vi "CODMn通讯.vi"() -> ()   [LabVIEW 2016, in "斯坦道CODMn.lvlib"]
uses:
  <vilib>/NI/Modbus Library/API/Wrapper/Create TCP Slave.vi
  <vilib>/NI/Modbus Library/API/slave/Modbus Slave.lvclass
  <vilib>/Plasmionique/MB Master/MB_Master/MB_Master.lvclass
  <vilib>/Plasmionique/MB Master/MB Master.lvlib
  <vilib>/NI/Modbus Library/API/Wrapper/API Main.lvlib
  <vilib>/ptbypt/NI_PtbyPt.lvlib
panel:
  out "F0-F5":u16[](array[numeric])
  out "codm程序更新":bool=TRUE
  in  "读取数据":bool
  in  "释放串口":bool
  in  "打开串口":bool
  out "队列中元素数量":i32
  out "元素":cluster{"命令":string}[](array[cluster])
  out "待处理插入数量":i32
  out "读取公式":u16[](array[numeric])
  out "读取参数":u16[](array[numeric])
  out "数据存储":u16[](array[numeric])
  out "温度":bool[](array[boolean])
  out "M输出点":bool[](array[boolean])
  out "ORP、时间":u16[](array[numeric])
  out "测量状态":u16[](array[numeric])
  out "通讯状态":bool
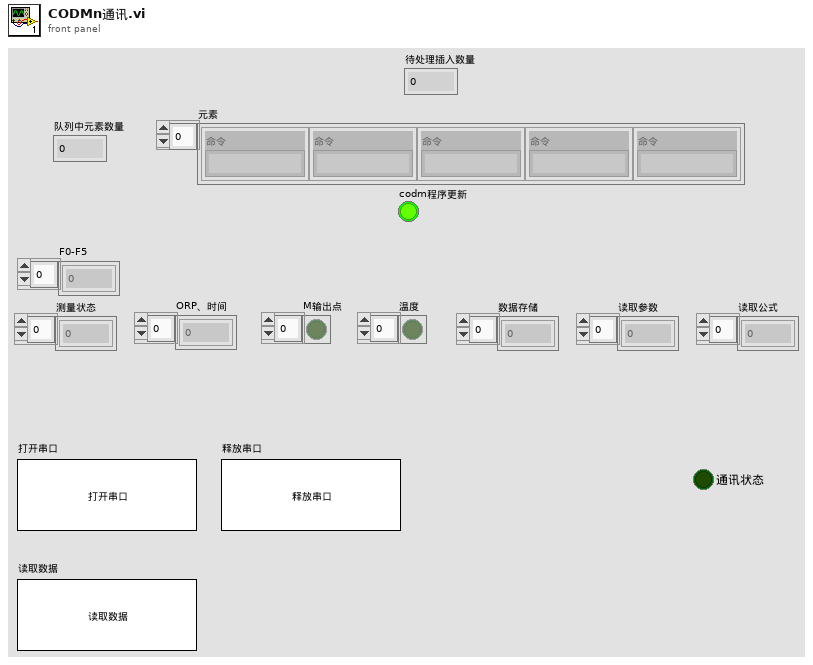
[diagram p1: front panel]
types:
  T1 = typedef "CODMn交互.ctl" = cluster{"COD浓度（mg/L)":dbl, "水样启动时间":timestamp, "加标回收启动时间":timestamp, "CODMn工作状态":enum16{"空闲", "水样测试", "标样核查", "零点核查", "跨度核查", "空白测试", "平行样测试", "加标回收", "空白校准", "标样校准", "初始化（清洗）"}, "多列列表框":i32, "平台试剂余量百分比":sgl, "关键参数":cluster{"测量量程":dbl, "测量精度":dbl, "测量间隔":dbl, "消解温度":dbl, "消解时长":dbl, "空白校准时间":timestamp, "曲线截距":dbl, "曲线斜率":dbl, "测量检出限":dbl, "测量信号值":dbl, "线性相关系数":dbl, "二次多项式系数":dbl, "标样校准时间":timestamp, "稀释倍数":dbl, "三项式系数":dbl, "空白标定系数":dbl, "量程系数":dbl, "F0/ORPA":dbl, "F1/ORPB":dbl, "F2/ORPK":dbl, "F3":dbl, "F4":dbl, "F5":dbl, "F6":dbl, "F7":dbl, "X0/滴定数":dbl, "量程":dbl}, "关键参数改变":bool, "校准信息":cluster{"低标液1浓度":dbl, "低标液1信号值":dbl, "低标液1启用":u16, "低标液2浓度":dbl, "低标液2信号值":dbl, "低标液2启用":u16, "低标液3浓度":dbl, "低标液3信号值":dbl, "低标液3启用":u16, "低标液4浓度":dbl, "低标液4信号值":dbl, "低标液4启用":u16, "低标液5浓度":dbl, "低标液5信号值":dbl, "低标液5启用":u16, "高标液1浓度":dbl, "高标液1信号值":dbl, "高标液1启用":u16, "高标液2浓度":dbl, "高标液2信号值":dbl, "高标液2启用":u16, "高标液3浓度":dbl, "高标液3信号值":dbl, "高标液3启用":u16, "高标液4浓度":dbl, "高标液4信号值":dbl, "高标液4启用":u16, "高标液5浓度":dbl, "高标液5信号值":dbl, "高标液5启用":u16}, "校准信息改变":bool}
  T2 = cluster{"测量模式":enum16{"水样测量", "标样核查", "零点核查", "跨度核查", "空白测试", "加标回收", "平行样", "校零", "校标"}}
  T3 = cluster{"命令":string, "测量模式":enum16{"水样测量", "标样核查", "零点核查", "跨度核查", "空白测试", "加标回收", "平行样", "校零", "校标"}, "CODMn量程切换":enum32{"H", "L", "AUTO"}}
  T4 = enum16{"空闲", "水样测试", "标样核查", "零点核查", "跨度核查", "空白测试", "平行样测试", "质控样", "空白校准", "标样校准", "加标回收"}
  T5 = cluster{"测量量程":dbl, "测量精度":dbl, "测量间隔":dbl, "消解温度":dbl, "消解时长":dbl, "空白校准时间":timestamp, "曲线截距":dbl, "曲线斜率":dbl, "测量检出限":dbl, "测量信号值":dbl, "线性相关系数":dbl, "二次多项式系数":dbl, "标样校准时间":timestamp, "稀释倍数":dbl, "三项式系数":dbl, "空白标定系数":dbl, "量程系数":dbl, "F0/ORPA":dbl, "F1/ORPB":dbl, "F2/ORPK":dbl, "F3":dbl, "F4":dbl, "F5":dbl, "F6":dbl, "F7":dbl, "X0/滴定数":dbl, "量程":dbl}
  T6 = enum16{"水样测量", "标样核查", "零点核查", "跨度核查", "空白测试", "加标回收", "平行样", "校零", "校标"}
  T7 = typedef "Alarm interface.lvlib/map in.ctl" = cluster{"name":string, "CN":string, "FirmwareVersion":string, "code":string}
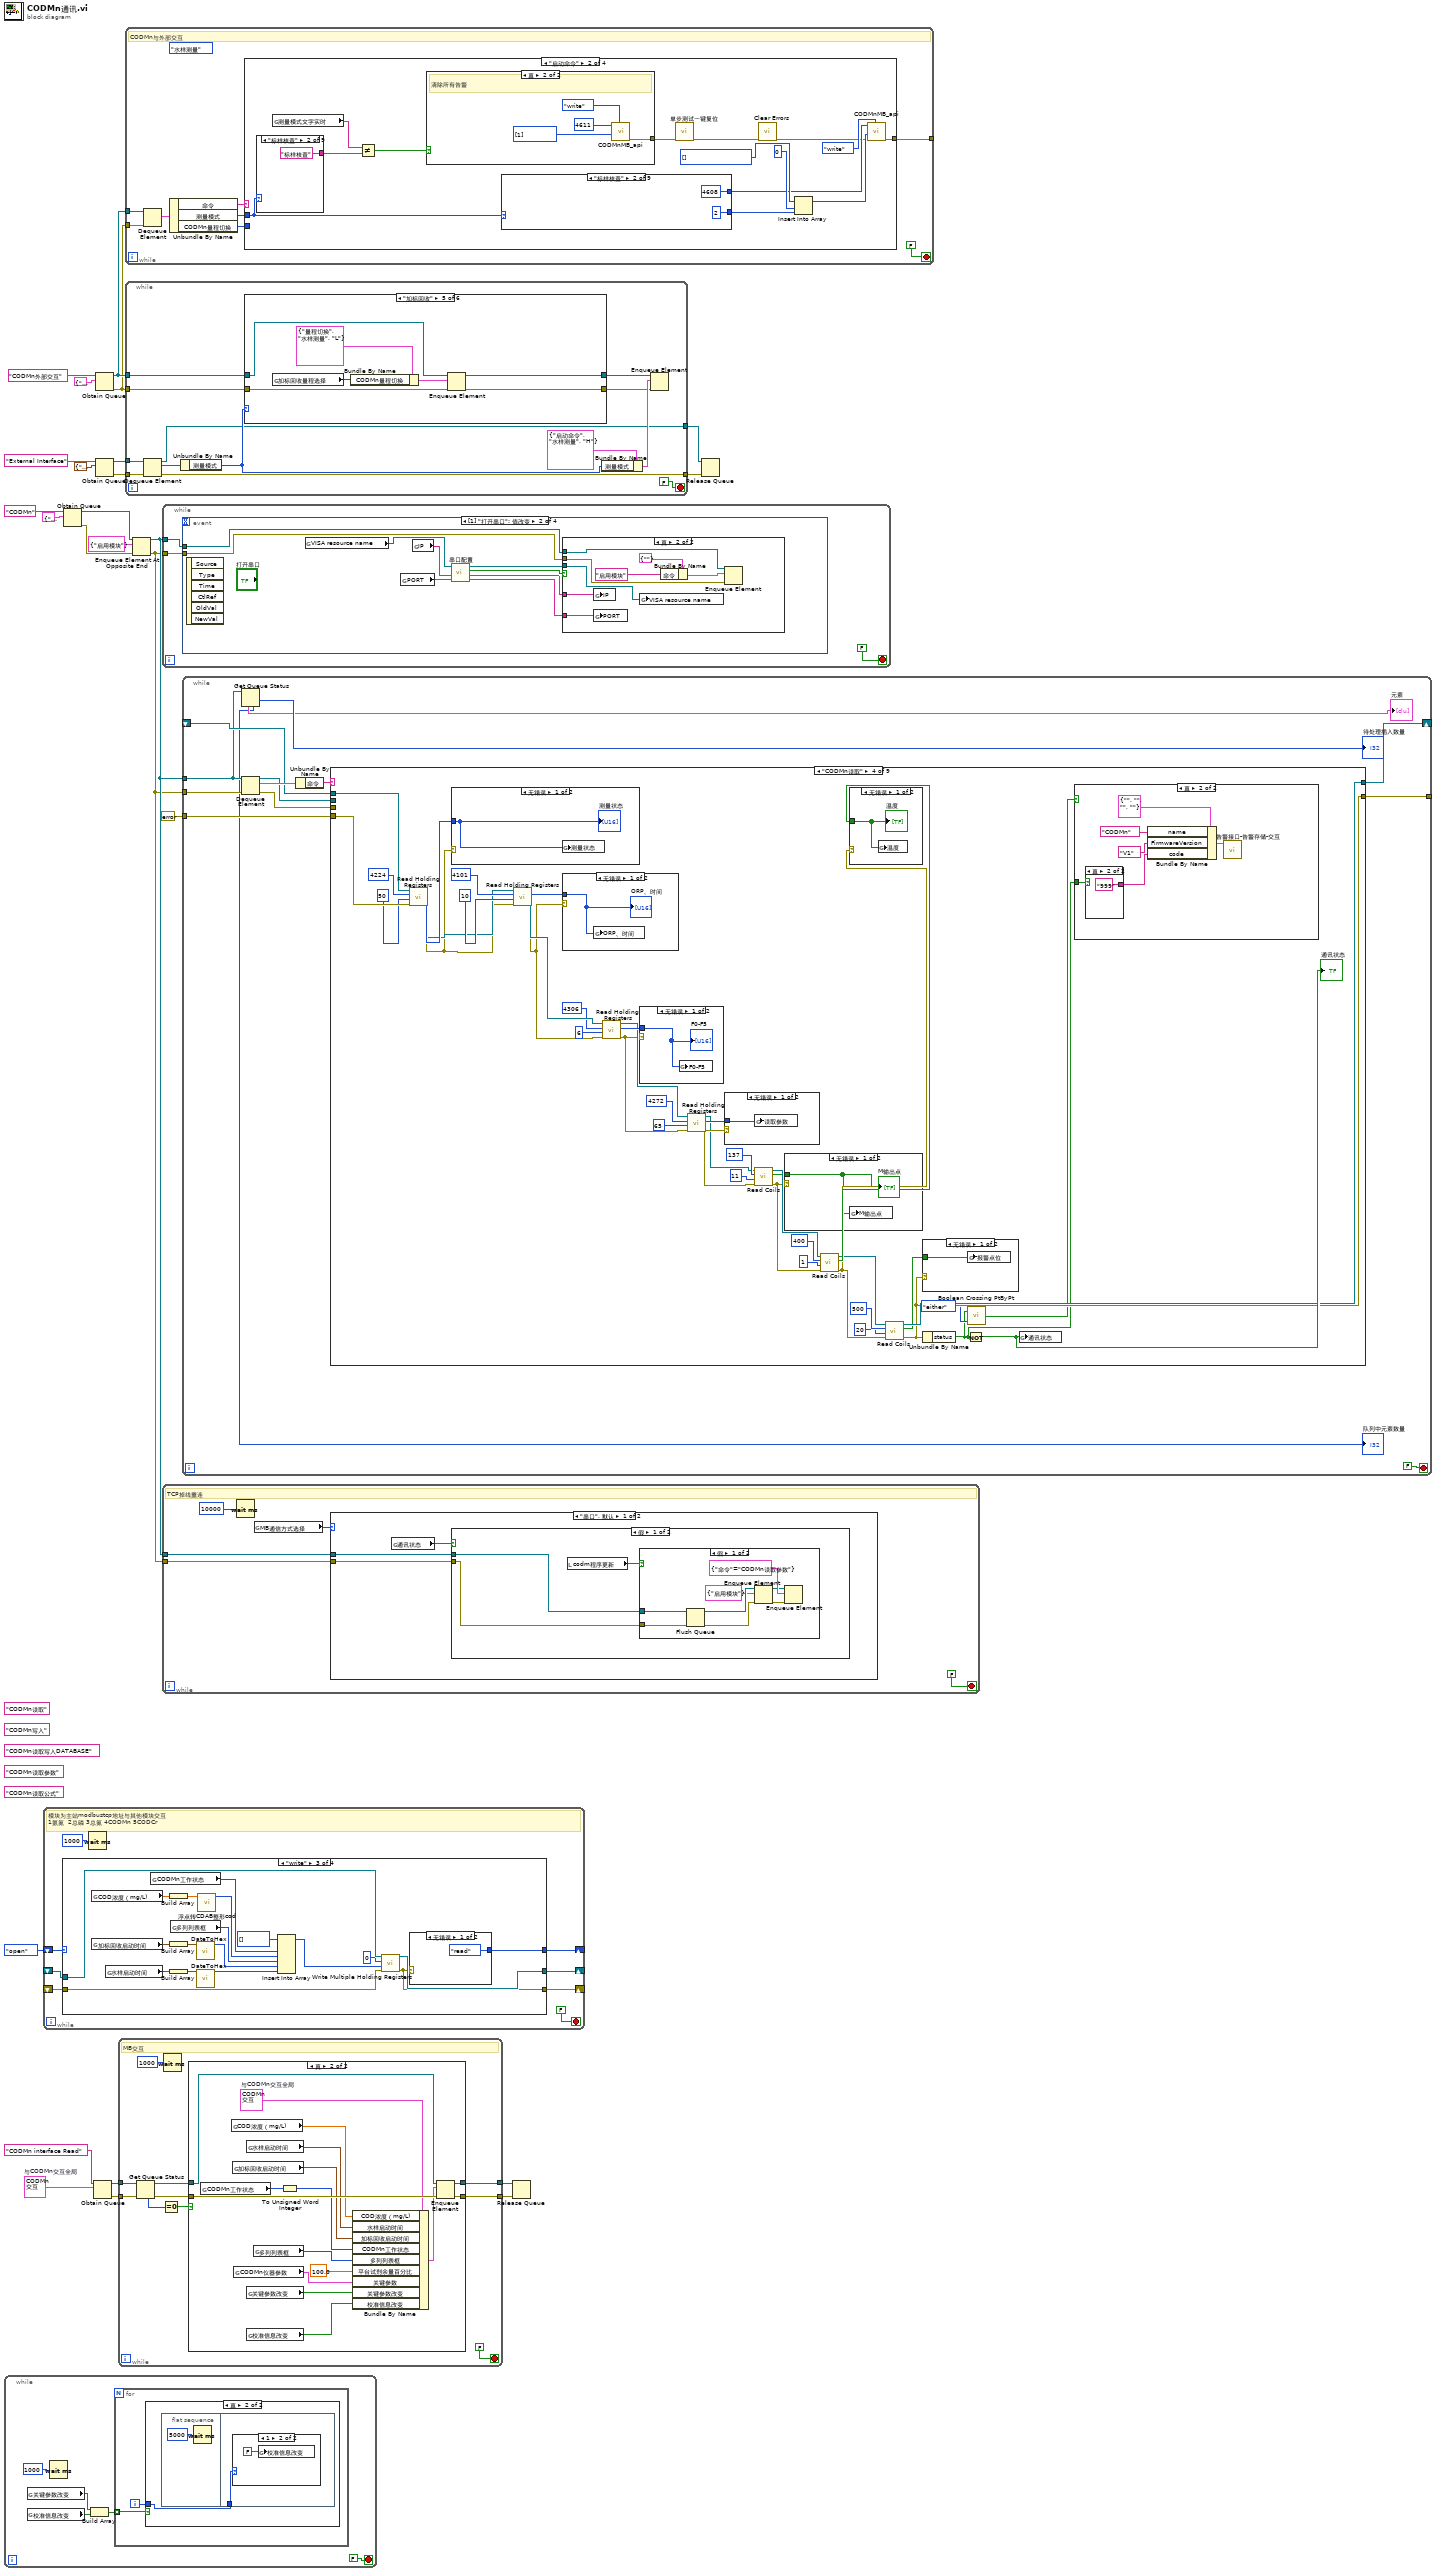
[diagram p0: block diagram]
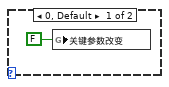
[diagram p3: hidden frame]
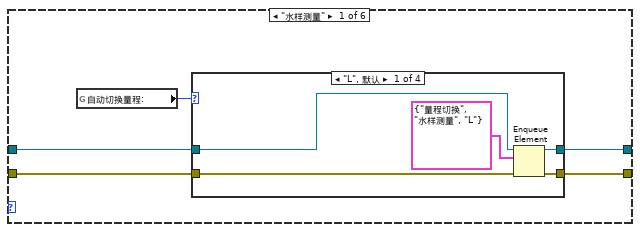
[diagram p5: hidden frame]
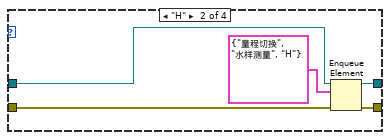
[diagram p6: hidden frame]
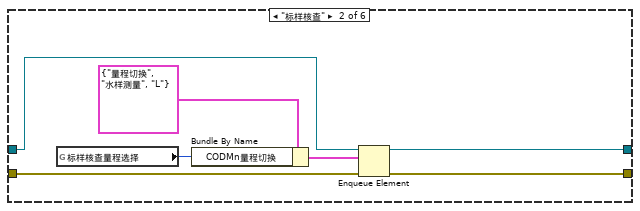
[diagram p9: hidden frame]
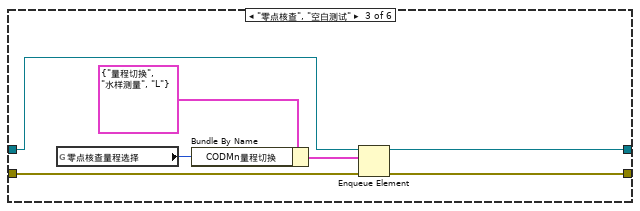
[diagram p10: hidden frame]
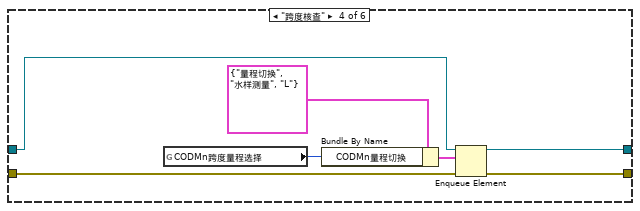
[diagram p11: hidden frame]
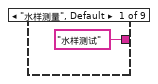
[diagram p15: hidden frame]
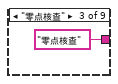
[diagram p16: hidden frame]
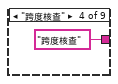
[diagram p17: hidden frame]
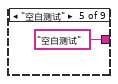
[diagram p18: hidden frame]
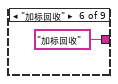
[diagram p19: hidden frame]
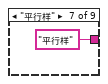
[diagram p20: hidden frame]
diagram:
  w2 = T1 {"COD浓度（mg/L)"=0.0, "水样启动时间"=timestamp(0 s since 1904-01-01), "加标回收启动时间"=timestamp(0 s since 1904-01-01), "CODMn工作状态"=enum."空闲", "多列列表框"=0, "平台试剂余量百分比"=0.0, "关键参数"={"测量量程"=0.0, "测量精度"=0.0, "测量间隔"=0.0, "消解温度"=0.0, "消解时长"=0.0, "空白校准时间"=timestamp(0 s since 1904-01-01), "曲线截距"=0.0, "曲线斜率"=0.0, "测量检出限"=0.0, "测量信号值"=0.0, "线性相关系数"=0.0, "二次多项式系数"=0.0, "标样校准时间"=timestamp(0 s since 1904-01-01), "稀释倍数"=0.0, "三项式系数"=0.0, "空白标定系数"=0.0, "量程系数"=0.0, "F0/ORPA"=0.0, "F1/ORPB"=0.0, "F2/ORPK"=0.0, "F3"=0.0, "F4"=0.0, "F5"=0.0, "F6"=0.0, "F7"=0.0, "X0/滴定数"=0.0, "量程"=0.0}, "关键参数改变"=FALSE, "校准信息"={"低标液1浓度"=0.0, "低标液1信号值"=0.0, "低标液1启用"=0, "低标液2浓度"=0.0, "低标液2信号值"=0.0, "低标液2启用"=0, "低标液3浓度"=0.0, "低标液3信号值"=0.0, "低标液3启用"=0, "低标液4浓度"=0.0, "低标液4信号值"=0.0, "低标液4启用"=0, "低标液5浓度"=0.0, "低标液5信号值"=0.0, "低标液5启用"=0, "高标液1浓度"=0.0, "高标液1信号值"=0.0, "高标液1启用"=0, "高标液2浓度"=0.0, "高标液2信号值"=0.0, "高标液2启用"=0, "高标液3浓度"=0.0, "高标液3信号值"=0.0, "高标液3启用"=0, "高标液4浓度"=0.0, "高标液4信号值"=0.0, "高标液4启用"=0, "高标液5浓度"=0.0, "高标液5信号值"=0.0, "高标液5启用"=0}, "校准信息改变"=FALSE}  # 与CODMn交互全局
  (unwired) "CODMn读取公式" ("名称（未命名）")
  (unwired) "CODMn读取写入DATABASE" ("名称（未命名）")
  (unwired) "CODMn读取参数" ("名称（未命名）")
  (unwired) "CODMn读取" ("名称（未命名）")
  (unwired) "CODMn写入" ("名称（未命名）")
  n1 = while {
    stop <- FALSE stop-if-true
    n2 = global read "CODMn断电保存全局变量.vi" "关键参数改变"() -> (w29:bool)
    n3 = global read "CODMn断电保存全局变量.vi" "校准信息改变"() -> (w28:bool)
    n4 = Wait (ms)(milliseconds to wait=u32 1000 ("等待时间（毫秒）")) -> ()  [unwired: 1 out]
    n5 = Build Array(w29, w28) -> (w27:bool[])
    n6 = for {
      tunnel: w27 -> [w32] mode=indexing
      i -> [w31]
      n7 = case shown="真" w32 {
        tunnel: w31 -> [_ w33]
        frame False {
        }
        frame True {
          n8 = flat-sequence {
            tunnel: w33 -> [w35]
            frame #0 {
              n9 = Wait (ms)(milliseconds to wait=u32 5000 ("等待时间（毫秒）")) -> ()  [unwired: 1 out]
            }
            frame #1 {
              n10 = case shown="1" w35 {
                frame 0, Default {
                  n11 = global write "CODMn断电保存全局变量.vi" "关键参数改变"(FALSE ("关键参数改变")) -> ()
                }
                frame 1 {
                  n12 = global write "CODMn断电保存全局变量.vi" "校准信息改变"(FALSE ("关键参数改变")) -> ()
                }
              }
            }
          }
        }
      }
    }
  }
  n13 = while {
    shift-right: [w43] -> _
    shift-left: _ -> [w45]
    shift-right: [w42] -> _
    shift-left: _ -> [w44]
    shift-right: [w39] -> _
    shift-left: enum16{"open", "read", "write", "close"}."open" -> [w40]
    stop <- FALSE stop-if-true
    # "模块为主站modbustcp地址与其他模块交互\n1氨氮  2总磷 3总氮 4CODMn 5CODCr"
    n14 = case shown="\"write\"" w40 {
      selector: w40 -> [w54 _ _ _]
      tunnel: w45 -> [w48 w62 w85 w91]
      tunnel: w44 -> [w47 w61 w82 w90]
      tunnel: [w51 w58 w84 w91] -> w43
      tunnel: [w50 w57 w83 w93] -> w42
      tunnel: [w53 w65 w86 enum16{"open", "read", "write", "close"}."open"] -> w39
      frame "open", Default {
        n15 = call-dynamic "Shutdown.vi"("error in"=w47, "Modbus slave in"=w48) -> ("error out"=w46:errorcluster)  [unwired: 9 in]
        n16 = call <vilib>:"Clear Errors.vi"("error in (no error)"=w46) -> ("error out"=w49:errorcluster)  [unwired: 5 in, 1 out]
        n17 = call-poly <vilib>:"Create Modbus Instance.vi"("error in"=w49, "port (502)"=u16 4) -> ("error out"=w50:errorcluster, "TCP slave instance"=w51:refnum<class "Modbus Slave.lvclass">)  [unwired: 8 in]
        n18 = case shown="错误" w50 {
          tunnel: w54 -> [_ w56]
          tunnel: [enum16{"open", "read", "write", "close"}."write" w56] -> w53
          frame No Error {
          }
          frame Error {
          }
        }
      }
      frame "read" {
        n19 = call-dynamic <vilib>:"Read Holding Registers.vi"("error in"=w61, "number of inputs"=u16 1, "starting address"=u16 257, "Modbus slave in"=w62) -> ("error out"=w57:errorcluster, "register values"=w60:u16[], "Modbus slave out"=w58:refnum<class "Modbus Slave.lvclass">)  [unwired: 5 in]
        n20 = case shown="无错误" w57 {
          tunnel: [enum16{"open", "read", "write", "close"}."write" enum16{"open", "read", "write", "close"}."close"] -> w65
          frame No Error {
          }
          frame Error {
          }
        }
        n21 = Index Array(array=w60) -> (element=w59:u16)  [unwired: 1 in]
        n22 = global write "CODMN外部API.vi" "CODMn状态"(w59) -> ()
      }
      frame "write" {
        n23 = global read "COD浓度全局变量.vi" "COD浓度（mg/L)"() -> (w74:dbl)
        n24 = global read "COD测量模式全局.vi" "加标回收启动时间"() -> (w77:timestamp)
        n25 = global read "COD测量模式全局.vi" "水样启动时间"() -> (w79:timestamp)
        n26 = global read "COD测量模式全局.vi" "CODMn工作状态"() -> (w72:T4)
        n27 = Build Array(w74) -> (w73:dbl[])
        n28 = Build Array(w77) -> (w70:timestamp[])
        n29 = Build Array(w79) -> (w78:timestamp[])
        n30 = global read "运行时序全局变量.vi" "多列列表框"() -> (w76:i32)
        n31 = call "DateToHex.vi"("DATE"=w70) -> ("数组"=w80:u16[])  [unwired: 10 in]
        n32 = call "DateToHex.vi"("DATE"=w78) -> ("数组"=w81:u16[])  [unwired: 10 in]
        n33 = call "浮点转CDAB整形cod.vi"("浮点数"=w73) -> ("CDAB整形输出"=w75:u16[])  [unwired: 10 in]
        n34 = Insert Into Array(array=u16[] [] ("values"), new element #1=w72, new element #2=w75, new element #3=w76, new element #4=w80, new element #5=w81) -> (w69:u16[])  [unwired: 1 in]
        n35 = call-dynamic "Write Multiple Holding Registers.vi"("error in"=w82, "registers to write"=w69, "starting address"=u16 0, "Modbus slave in"=w85) -> ("error out"=w83:errorcluster, "Modbus slave out"=w84:refnum<class "Modbus Slave.lvclass">)  [unwired: 6 in]
        n36 = case shown="无错误" w83 {
          tunnel: [enum16{"open", "read", "write", "close"}."read" enum16{"open", "read", "write", "close"}."close"] -> w86
          frame No Error {
          }
          frame Error {
          }
        }
      }
      frame "close" {
        n37 = call-dynamic "Shutdown.vi"("error in"=w90, "Modbus slave in"=w91) -> ("error out"=w89:errorcluster)  [unwired: 9 in]
        n38 = call <vilib>:"Clear Errors.vi"("error in (no error)"=w89) -> ("error out"=w93:errorcluster)  [unwired: 5 in, 1 out]
      }
    }
    n39 = Wait (ms)(milliseconds to wait=u32 1000 ("等待时间（毫秒）")) -> ()  [unwired: 1 out]
  }
  n40 = Obtain Queue(name (unnamed)="CODMn", element data type=cluster{"命令":string} {"命令"="启用模块"} ("元素")) -> (queue out=w23:refnum<queue>, error out=w22:errorcluster)  [unwired: 3 in, 1 out]
  n41 = Obtain Queue(name (unnamed)="CODMn interface Read" ("写入方名称"), element data type=w2) -> (queue out=w6:refnum<queue>, error out=w5:errorcluster)  [unwired: 3 in, 1 out]
  n42 = Obtain Queue(name (unnamed)="CODMn外部交互" ("名称（未命名）"), element data type=T3 {"命令"="启动命令", "测量模式"=enum."水样测量", "CODMn量程切换"=enum."AUTO"} ("元素")) -> (queue out=w11:refnum<queue>, error out=w10:errorcluster)  [unwired: 3 in, 1 out]
  n43 = Obtain Queue(name (unnamed)="External Interface" ("名称（未命名）"), element data type=T2 {"测量模式"=enum."水样测量"} ("启动测量模式")) -> (queue out=w13:refnum<queue>, error out=w12:errorcluster)  [unwired: 3 in, 1 out]
  n44 = while {
    tunnel: w6 -> [w102]
    tunnel: w5 -> [w95]
    tunnel: [w101] -> w4
    tunnel: [w100] -> w3
    stop <- FALSE stop-if-true
    # "MB交互"
    n45 = Get Queue Status(queue=w102, error in (no error)=w95) -> (queue out=w98:refnum<queue>, error out=w94:errorcluster, # elements in queue=w97:i32)  [unwired: 1 in, 5 out]
    n46 = Equal To 0?(x=w97) -> (x = 0?=w96:bool)
    n47 = Wait (ms)(milliseconds to wait=u32 1000 ("等待时间（毫秒）")) -> ()  [unwired: 1 out]
    n48 = case shown="真" w96 {
      tunnel: w98 -> [w105 w121]
      tunnel: w94 -> [w104 w120]
      tunnel: [w105 w119] -> w101
      tunnel: [w104 w118] -> w100
      frame False {
      }
      frame True {
        w117 = T1 {"COD浓度（mg/L)"=0.0, "水样启动时间"=timestamp(0 s since 1904-01-01), "加标回收启动时间"=timestamp(0 s since 1904-01-01), "CODMn工作状态"=enum."空闲", "多列列表框"=0, "平台试剂余量百分比"=0.0, "关键参数"={"测量量程"=0.0, "测量精度"=0.0, "测量间隔"=0.0, "消解温度"=0.0, "消解时长"=0.0, "空白校准时间"=timestamp(0 s since 1904-01-01), "曲线截距"=0.0, "曲线斜率"=0.0, "测量检出限"=0.0, "测量信号值"=0.0, "线性相关系数"=0.0, "二次多项式系数"=0.0, "标样校准时间"=timestamp(0 s since 1904-01-01), "稀释倍数"=0.0, "三项式系数"=0.0, "空白标定系数"=0.0, "量程系数"=0.0, "F0/ORPA"=0.0, "F1/ORPB"=0.0, "F2/ORPK"=0.0, "F3"=0.0, "F4"=0.0, "F5"=0.0, "F6"=0.0, "F7"=0.0, "X0/滴定数"=0.0, "量程"=0.0}, "关键参数改变"=FALSE, "校准信息"={"低标液1浓度"=0.0, "低标液1信号值"=0.0, "低标液1启用"=0, "低标液2浓度"=0.0, "低标液2信号值"=0.0, "低标液2启用"=0, "低标液3浓度"=0.0, "低标液3信号值"=0.0, "低标液3启用"=0, "低标液4浓度"=0.0, "低标液4信号值"=0.0, "低标液4启用"=0, "低标液5浓度"=0.0, "低标液5信号值"=0.0, "低标液5启用"=0, "高标液1浓度"=0.0, "高标液1信号值"=0.0, "高标液1启用"=0, "高标液2浓度"=0.0, "高标液2信号值"=0.0, "高标液2启用"=0, "高标液3浓度"=0.0, "高标液3信号值"=0.0, "高标液3启用"=0, "高标液4浓度"=0.0, "高标液4信号值"=0.0, "高标液4启用"=0, "高标液5浓度"=0.0, "高标液5信号值"=0.0, "高标液5启用"=0}, "校准信息改变"=FALSE}  # 与CODMn交互全局
        n49 = global read "COD测量模式全局.vi" "CODMn工作状态"() -> (w114:T4)
        n50 = global read "COD浓度全局变量.vi" "COD浓度（mg/L)"() -> (w109:dbl)
        n51 = global read "COD测量模式全局.vi" "加标回收启动时间"() -> (w113:timestamp)
        n52 = global read "CODMn断电保存全局变量.vi" "CODMn仪器参数"() -> (w116:T5)
        n53 = global read "COD测量模式全局.vi" "水样启动时间"() -> (w112:timestamp)
        n54 = global read "CODMn断电保存全局变量.vi" "关键参数改变"() -> (w107:bool)
        n55 = global read "CODMn断电保存全局变量.vi" "校准信息改变"() -> (w106:bool)
        n56 = global read "运行时序全局变量.vi" "多列列表框"() -> (w110:i32)
        n57 = To Unsigned Word Integer(number=w114) -> (unsigned 16bit integer=w115:u16)
        n58 = Bundle By Name(cluster=w117, "COD浓度（mg/L)"=w109, "水样启动时间"=w112, "加标回收启动时间"=w113, "CODMn工作状态"=w115, "多列列表框"=w110, "平台试剂余量百分比"=sgl 100.0, "关键参数"=w116, "关键参数改变"=w107, "校准信息改变"=w106) -> (w108:T1)
        n59 = Enqueue Element(queue=w121, element=w108, error in (no error)=w120) -> (queue out=w119:refnum<queue>, error out=w118:errorcluster)  [unwired: 1 in, 1 out]
      }
    }
  }
  n60 = while {
    tunnel: w11 -> [w127]
    tunnel: w10 -> [w126]
    tunnel: [w122] -> _
    stop <- FALSE stop-if-true
    (unwired) T6."水样测量" ("测量模式")
    # "CODMn与外部交互"
    n61 = Dequeue Element(queue=w127, error in (no error)=w126) -> (element=w128:T3)  [unwired: 1 in, 3 out]
    n62 = Unbundle By Name(w128) -> ("命令"=w125:string, "测量模式"=w124:T6, "CODMn量程切换"=w123:enum32{"H", "L", "AUTO"})
    n63 = case shown="\"启动命令\"" w125 {
      tunnel: w124 -> [_ w132 _ _]
      tunnel: w123 -> [_ _ _ w182]
      tunnel: [_ w137 w177 w181] -> w122
      frame "假", Default {
      }
      frame "启动命令" {
        n64 = case shown="\"标样核查\"" w132 {
          tunnel: ["水样测试" ("测量模式") "标样核查" ("测量模式") "零点核查" ("测量模式") "跨度核查" ("测量模式") "空白测试" ("测量模式") "加标回收" ("测量模式") "平行样" ("测量模式") "校零" ("测量模式") "校标" ("测量模式")] -> w134
          frame "水样测量", Default {
          }
          frame "标样核查" {
          }
          frame "零点核查" {
          }
          frame "跨度核查" {
          }
          frame "空白测试" {
          }
          frame "加标回收" {
          }
          frame "平行样" {
          }
          frame "校零" {
          }
          frame "校标" {
          }
        }
        n65 = global read "COD测量模式全局.vi" "测量模式文字实时"() -> (w133:string)
        n66 = Not Equal?(x=w133, y=w134) -> (x != y?=w131:bool)
        n67 = case shown="真" w131 {
          tunnel: [_ w144] -> w130
          frame False {
          }
          frame True {
            # "清除所有告警"
            n68 = call "CODMnMB_api.vi"("STEP"=enum16{"open", "read", "write", "close"}."write", "values"=u16[] [1], "starting address"=u16 4611) -> ("error out"=w144:errorcluster)  [unwired: 6 in, 2 out]
          }
        }
        n69 = case shown="\"标样核查\"" w132 {
          tunnel: [u16 4608 ("address") u16 4608 ("address") u16 4608 ("address") u16 4608 ("address") u16 4608 ("address") u16 4608 ("address") u16 4608 ("address") u16 4608 ("address") u16 4608 ("address")] -> w139
          tunnel: [u16 1 ("address") u16 2 ("address") u16 3 ("address") u16 4 ("address") u16 5 ("address") u16 7 ("address") u16 6 ("address") u16 8 ("address") u16 9 ("address")] -> w143
          frame "水样测量" {
          }
          frame "标样核查" {
          }
          frame "零点核查" {
          }
          frame "跨度核查" {
          }
          frame "空白测试" {
          }
          frame "加标回收" {
          }
          frame "平行样" {
          }
          frame "校零" {
            n70 = global write "CODMN外部API.vi" "远程反控校零CODMn"(TRUE ("远程反控校准CODMn")) -> ()
          }
          frame "校标" {
            n71 = global write "CODMN外部API.vi" "远程反控校准CODMn"(TRUE ("远程反控校准CODMn")) -> ()
          }
        }
        n72 = call "单步测试一键复位.vi"("Error in"=w130) -> ("error out"=w136:errorcluster)  [unwired: 10 in]
        n73 = call <vilib>:"Clear Errors.vi"("error in (no error)"=w136) -> ("error out"=w135:errorcluster)  [unwired: 5 in, 1 out]
        n74 = Insert Into Array(array=u16[] [] ("values"), index=0 ("索引"), new element=w143) -> (w138:u16[])
        n75 = call "CODMnMB_api.vi"("STEP"=enum16{"open", "read", "write", "close"}."write", "Error in"=w135, "values"=w138, "starting address"=w139) -> ("error out"=w137:errorcluster)  [unwired: 5 in, 2 out]
      }
      frame "停止命令" {
        n76 = call "CODMnMB_api.vi"("STEP"=enum16{"open", "read", "write", "close"}."write", "values"=u16[] [11], "starting address"=u16 4608) -> ("error out"=w177:errorcluster)  [unwired: 6 in, 2 out]
      }
      frame "量程切换" {
        n77 = case shown="\"H\"" w182 {
          tunnel: [u16[] [1] ("values") u16[] [0] ("values") _] -> w185
          frame "H" {
          }
          frame "L" {
          }
          frame "AUTO", Default {
          }
        }
        n78 = call "CODMnMB_api.vi"("STEP"=enum16{"open", "read", "write", "close"}."write", "values"=w185, "starting address"=u16 4276) -> ("error out"=w181:errorcluster)  [unwired: 6 in, 2 out]
      }
    }
  }
  n79 = while {
    tunnel: w13 -> [w200]
    tunnel: w12 -> [w199]
    tunnel: w11 -> [w196]
    tunnel: w10 -> [w195]
    tunnel: [w189] -> w9
    tunnel: [w188] -> w8
    stop <- FALSE stop-if-true
    n80 = Dequeue Element(queue=w200, error in (no error)=w199) -> (queue out=w189:refnum<queue>, element=w197:T2, error out=w188:errorcluster)  [unwired: 1 in, 1 out]
    n81 = Unbundle By Name(w197) -> ("测量模式"=w192:T6)
    n82 = case "条件结构" shown="\"加标回收\"" w192 {
      tunnel: w196 -> [w204 w223 w230 w237 w244 w249]
      tunnel: w195 -> [w202 w222 w229 w236 w243 w248]
      tunnel: [w203 w221 w228 w235 w242 w249] -> w191
      tunnel: [w201 w220 w227 w234 w241 w248] -> w190
      frame "水样测量" {
        n83 = global read "CODMn断电保存全局变量.vi" "自动切换量程:"() -> (w205:enum16{"L", "H", "自动切换测一次", "自动切换测两次"})
        n84 = case shown="\"L\", 默认" w205 {
          tunnel: w204 -> [w209 w215 w216 w219]
          tunnel: [w207 w214 w216 w219] -> w203
          tunnel: w202 -> [w208 w213 w217 w218]
          tunnel: [w206 w212 w217 w218] -> w201
          frame "L", Default {
            n85 = Enqueue Element(queue=w209, element=T3 {"命令"="量程切换", "测量模式"=enum."水样测量", "CODMn量程切换"=enum."L"} ("元素"), error in (no error)=w208) -> (queue out=w207:refnum<queue>, error out=w206:errorcluster)  [unwired: 1 in, 1 out]
          }
          frame "H" {
            n86 = Enqueue Element(queue=w215, element=T3 {"命令"="量程切换", "测量模式"=enum."水样测量", "CODMn量程切换"=enum."H"} ("元素"), error in (no error)=w213) -> (queue out=w214:refnum<queue>, error out=w212:errorcluster)  [unwired: 1 in, 1 out]
          }
          frame "自动切换测一次" {
          }
          frame "自动切换测两次" {
          }
        }
      }
      frame "标样核查" {
        n87 = global read "CODMn断电保存全局变量.vi" "标样核查量程选择"() -> (w225:enum32{"H", "L", "AUTO"})
        n88 = Bundle By Name(cluster=T3 {"命令"="量程切换", "测量模式"=enum."水样测量", "CODMn量程切换"=enum."L"} ("元素"), "CODMn量程切换"=w225) -> (w226:T3)
        n89 = Enqueue Element(queue=w223, element=w226, error in (no error)=w222) -> (queue out=w221:refnum<queue>, error out=w220:errorcluster)  [unwired: 1 in, 1 out]
      }
      frame "零点核查", "空白测试" {
        n90 = global read "CODMn断电保存全局变量.vi" "零点核查量程选择"() -> (w232:enum32{"H", "L", "AUTO"})
        n91 = Bundle By Name(cluster=T3 {"命令"="量程切换", "测量模式"=enum."水样测量", "CODMn量程切换"=enum."L"} ("元素"), "CODMn量程切换"=w232) -> (w231:T3)
        n92 = Enqueue Element(queue=w230, element=w231, error in (no error)=w229) -> (queue out=w228:refnum<queue>, error out=w227:errorcluster)  [unwired: 1 in, 1 out]
      }
      frame "跨度核查" {
        n93 = global read "CODMn断电保存全局变量.vi" "CODMn跨度量程选择"() -> (w239:enum32{"H", "L", "AUTO"})
        n94 = Bundle By Name(cluster=T3 {"命令"="量程切换", "测量模式"=enum."水样测量", "CODMn量程切换"=enum."L"} ("元素"), "CODMn量程切换"=w239) -> (w238:T3)
        n95 = Enqueue Element(queue=w237, element=w238, error in (no error)=w236) -> (queue out=w235:refnum<queue>, error out=w234:errorcluster)  [unwired: 1 in, 1 out]
      }
      frame "加标回收" {
        n96 = global read "CODMn断电保存全局变量.vi" "加标回收量程选择"() -> (w246:enum32{"H", "L", "AUTO"})
        n97 = Bundle By Name(cluster=T3 {"命令"="量程切换", "测量模式"=enum."水样测量", "CODMn量程切换"=enum."L"} ("元素"), "CODMn量程切换"=w246) -> (w245:T3)
        n98 = Enqueue Element(queue=w244, element=w245, error in (no error)=w243) -> (queue out=w242:refnum<queue>, error out=w241:errorcluster)  [unwired: 1 in, 1 out]
      }
      frame Default {
        # "不切换量程"
      }
    }
    n99 = Bundle By Name(cluster=T3 {"命令"="启动命令", "测量模式"=enum."水样测量", "CODMn量程切换"=enum."H"} ("元素"), "测量模式"=w192) -> (w193:T3)
    n100 = Enqueue Element(queue=w191, element=w193, error in (no error)=w190) -> ()  [unwired: 1 in, 3 out]
  }
  n101 = Enqueue Element At Opposite End(queue=w23, element=cluster{"命令":string} {"命令"="启用模块"} ("元素"), error in (no error)=w22) -> (queue out=w19:refnum<queue>, error out=w18:errorcluster)  [unwired: 1 in, 1 out]
  n102 = while {
    tunnel: w19 -> [w251]
    tunnel: w18 -> [w250]
    stop <- FALSE stop-if-true
    n103 = event shown="[1] \"打开串口\": 值改变" {
      selector: _ -> [_ _ _ _]
      dyn-events: _ -> [_ _ _ _]
      timeout: _ -> [_ _ _ _]
      tunnel: w251 -> [_ w258 w272 w274]
      tunnel: w250 -> [_ w257 w271 w273]
      event Timeout {
        n104 = event-data() -> ()  [unwired: 1 in, 3 out]
      }
      event "打开串口": Value Change {
        n105 = event-data() -> ()  [unwired: 1 in, 6 out]
        n106 = global read "CODMn断电保存全局变量.vi" "VISA resource name"() -> (w261:refnum<visa-resource-name>)
        n107 = global read "CODMn断电保存全局变量.vi" "PORT"() -> (w253:string)
        n108 = global read "CODMn断电保存全局变量.vi" "IP"() -> (w254:string)
        n109 = call "串口配置.vi"("PORT"=w253, "IP"=w254, "请选择串口:"=w261) -> ("PORT 2"=w255:string, "IP 2"=w256:string, "确认 2"=w259:bool, "VISA资源名称 2"=w260:refnum<visa-resource-name>)  [unwired: 4 in, 1 out]
        n110 = case shown="真" w259 {
          tunnel: w260 -> [_ w269]
          tunnel: w258 -> [_ w265]
          tunnel: w257 -> [_ w264]
          tunnel: w256 -> [_ w263]
          tunnel: w255 -> [_ w262]
          frame False {
          }
          frame True {
            n111 = global write "CODMn断电保存全局变量.vi" "IP"(w263) -> ()
            n112 = global write "CODMn断电保存全局变量.vi" "PORT"(w262) -> ()
            n113 = global write "CODMn断电保存全局变量.vi" "VISA resource name"(w269) -> ()
            n114 = Bundle By Name(cluster=cluster{"命令":string} {"命令"=""} ("元素"), "命令"="启用模块" ("名称（未命名）")) -> (w266:cluster{"命令":string})
            n115 = Enqueue Element(queue=w265, element=w266, error in (no error)=w264) -> ()  [unwired: 1 in, 3 out]
          }
        }
      }
      event "释放串口": Value Change {
        n116 = event-data() -> ()  [unwired: 1 in, 6 out]
        n117 = Enqueue Element(queue=w272, element=cluster{"命令":string} {"命令"="停用模块"} ("元素"), error in (no error)=w271) -> ()  [unwired: 1 in, 3 out]
      }
      event "读取数据": Value Change {
        n118 = event-data() -> ()  [unwired: 1 in, 6 out]
        n119 = Enqueue Element(queue=w274, element=cluster{"命令":string} {"命令"="CODMn读取"} ("元素"), error in (no error)=w273) -> ()  [unwired: 1 in, 3 out]
      }
    }
  }
  n120 = while "While循环" {
    tunnel: w19 -> [w277]
    tunnel: w18 -> [w276]
    stop <- FALSE stop-if-true
    # "TCP掉线重连"
    n121 = Wait (ms)(milliseconds to wait=u32 10000 ("等待时间（毫秒）")) -> ()  [unwired: 1 out]
    n122 = global read "CODMn断电保存全局变量.vi" "MB通信方式选择"() -> (w278:enum16{"串口", "TCP"})
    n123 = case shown="\"串口\", 默认" w278 {
      tunnel: w277 -> [w282 w296]
      tunnel: w276 -> [w281 w295]
      frame "串口", Default {
        n124 = global read "COD内部交互全局.vi" "通讯状态"() -> (w283:bool)
        n125 = case shown="假" w283 {
          tunnel: w282 -> [w286 _]
          tunnel: w281 -> [w285 _]
          frame False {
            n126 = local read "codm程序更新"() -> (w284:bool)
            n127 = case shown="假" w284 {
              tunnel: w286 -> [w291 _]
              tunnel: w285 -> [w290 _]
              frame False {
                n128 = Flush Queue(queue=w291, error in (no error)=w290) -> (queue out=w294:refnum<queue>, error out=w293:errorcluster)  [unwired: 1 out]
                n129 = Enqueue Element(queue=w294, element=cluster{"命令":string} {"命令"="启用模块"} ("元素"), error in (no error)=w293) -> (queue out=w288:refnum<queue>, error out=w287:errorcluster)  [unwired: 1 in, 1 out]
                n130 = Enqueue Element(queue=w288, element=cluster{"命令":string} {"命令"="CODMn读取参数"} ("元素"), error in (no error)=w287) -> ()  [unwired: 1 in, 3 out]
              }
              frame True {
              }
            }
          }
          frame True {
          }
        }
      }
      frame "TCP" {
        n131 = global read "COD浓度全局变量.vi" "MB session in"() -> (w298:refnum<class "MB_Master.lvclass">)
        n132 = property class="MB_Master"(reference=w298) -> ("Properties:Session Valid"=w297:bool)  [unwired: 1 in, 2 out]
        n133 = case shown="假" w297 {
          tunnel: w296 -> [w303 _]
          tunnel: w295 -> [w302 _]
          frame False {
            n134 = Flush Queue(queue=w303, error in (no error)=w302) -> (queue out=w306:refnum<queue>, error out=w305:errorcluster)  [unwired: 1 out]
            n135 = Enqueue Element(queue=w306, element=cluster{"命令":string} {"命令"="启用模块"} ("元素"), error in (no error)=w305) -> (queue out=w300:refnum<queue>, error out=w299:errorcluster)  [unwired: 1 in, 1 out]
            n136 = Enqueue Element(queue=w300, element=cluster{"命令":string} {"命令"="CODMn读取参数"} ("元素"), error in (no error)=w299) -> ()  [unwired: 1 in, 3 out]
          }
          frame True {
          }
        }
      }
    }
  }
  n137 = while {
    tunnel: w19 -> [w312]
    tunnel: w18 -> [w319]
    tunnel: [w313] -> _
    shift-right: [w316] -> _
    shift-left: _ -> [w315]
    tunnel: errorcluster {"status"=FALSE, "code"=0, "source"=""} ("error out") -> [w314]
    stop <- FALSE stop-if-true
    n138 = Get Queue Status(queue=w312) -> (# pending insert=→"待处理插入数量":i32, # elements in queue=→"队列中元素数量":i32, elements=→"元素":cluster{"命令":string}[])  [unwired: 2 in, 5 out]
    n139 = Dequeue Element(queue=w312, error in (no error)=w319) -> (queue out=w308:refnum<queue>, element=w318:cluster{"命令":string}, error out=w307:errorcluster)  [unwired: 1 in, 1 out]
    n140 = Unbundle By Name(w318) -> ("命令"=w317:string)
    n141 = case shown="\"CODMn读取\"" w317 {
      tunnel: [w322 w327 w339 w362 w401 w410 w427 w434 w441] -> w316
      tunnel: [w321 w324 w340 w359 w399 w409 w426 w433 w440] -> w313
      tunnel: w315 -> [w322 _ _ w383 w405 w419 w430 w438 w444]
      tunnel: w314 -> [w321 w328 w341 w382 w402 w418 w429 w437 w442]
      tunnel: w308 -> [_ w326 _ _ _ _ _ _ _]
      tunnel: w307 -> [_ w325 _ _ _ _ _ _ _]
      frame Default {
      }
      frame "启用模块" {
        n142 = local write "codm程序更新"(FALSE ("codm程序更新")) -> ()
        n143 = call "CODMnMB_api.vi"("STEP"=enum16{"open", "read", "write", "close"}."open", "Error in"=w328) -> ("error out"=w324:errorcluster, "MB session out"=w327:refnum<class "MB_Master.lvclass">)  [unwired: 7 in, 1 out]
        n144 = case shown="无错误" w324 {
          tunnel: w326 -> [w334 _]
          tunnel: w325 -> [w333 _]
          frame No Error {
            n145 = global read "COD内部交互全局.vi" "序列号:"() -> (w332:string)
            n146 = Empty String/Path?(string/path=w332) -> (empty?=w331:bool)
            n147 = Not(x=w331) -> (.not. x?=w330:bool)
            n148 = case shown="真" w330 {
              tunnel: w334 -> [_ w337]
              tunnel: w333 -> [_ w336]
              frame False {
              }
              frame True {
                # "发货调试版用"
                n149 = Enqueue Element(queue=w337, element=cluster{"命令":string} {"命令"="CODMn序列号写入"} ("元素"), error in (no error)=w336) -> ()  [unwired: 1 in, 3 out]
              }
            }
          }
          frame Error {
          }
        }
        n150 = global write "COD浓度全局变量.vi" "MB session in"(w327) -> ()
      }
      frame "停用模块" {
        n151 = call "CODMnMB_api.vi"("STEP"=enum16{"open", "read", "write", "close"}."close", "Error in"=w341) -> ("error out"=w340:errorcluster, "MB session out"=w339:refnum<class "MB_Master.lvclass">)  [unwired: 7 in, 1 out]
        "codm程序更新" <- TRUE
      }
      frame "CODMn读取" {
        n152 = call <vilib>:"Read Holding Registers.vi"("error in (no error)"=w382, "quantity"=u16 50 ("number of holding registers"), "starting address"=u16 4224, "MB session in"=w383) -> ("error out"=w373:errorcluster, "Registers"=w379:u16[], "MB session out"=w374:refnum<class "MB_Master.lvclass">)  [unwired: 5 in]
        n153 = case shown="无错误" w373 {
          tunnel: w379 -> [w398 _]
          frame No Error {
            n154 = global write "COD内部交互全局.vi" "测量状态"(w398) -> ()
            "测量状态" <- w398
          }
          frame Error {
          }
        }
        n155 = call <vilib>:"Read Holding Registers.vi"("error in (no error)"=w373, "quantity"=u16 10, "starting address"=u16 4101, "MB session in"=w374) -> ("error out"=w356:errorcluster, "Registers"=w372:u16[], "MB session out"=w357:refnum<class "MB_Master.lvclass">)  [unwired: 5 in]
        n156 = case shown="无错误" w356 {
          tunnel: w372 -> [w397 _]
          frame No Error {
            n157 = global write "COD内部交互全局.vi" "ORP、时间"(w397) -> ()
            "ORP、时间" <- w397
          }
          frame Error {
          }
        }
        n158 = call <vilib>:"Read Holding Registers.vi"("error in (no error)"=w356, "quantity"=u16 6 ("number of holding registers"), "starting address"=u16 4306, "MB session in"=w357) -> ("error out"=w348:errorcluster, "Registers"=w353:u16[], "MB session out"=w349:refnum<class "MB_Master.lvclass">)  [unwired: 5 in]
        n159 = case shown="无错误" w348 {
          tunnel: w353 -> [w393 _]
          frame No Error {
            n160 = global write "COD内部交互全局.vi" "F0-F5"(w393) -> ()
            "F0-F5" <- w393
          }
          frame Error {
          }
        }
        n161 = call <vilib>:"Read Holding Registers.vi"("error in (no error)"=w348, "quantity"=u16 65 ("number of holding registers"), "starting address"=u16 4272, "MB session in"=w349) -> ("error out"=w347:errorcluster, "Registers"=w352:u16[], "MB session out"=w346:refnum<class "MB_Master.lvclass">)  [unwired: 5 in]
        n162 = case shown="无错误" w347 {
          tunnel: w352 -> [w392 _]
          frame No Error {
            n163 = global write "COD内部交互全局.vi" "读取参数"(w392) -> ()
          }
          frame Error {
          }
        }
        n164 = call <vilib>:"Read Coils.vi"("error in (no error)"=w347, "quantity"=u16 11, "starting address"=u16 137, "MB session in"=w346) -> ("error out"=w369:errorcluster, "Coils"=w370:bool[], "MB session out"=w371:refnum<class "MB_Master.lvclass">)  [unwired: 5 in]
        n165 = case shown="无错误" w369 {
          tunnel: w370 -> [w396 _]
          frame No Error {
            n166 = global write "COD内部交互全局.vi" "M输出点"(w396) -> ()
            "M输出点" <- w396
          }
          frame Error {
          }
        }
        n167 = call <vilib>:"Read Coils.vi"("error in (no error)"=w369, "quantity"=u16 1, "starting address"=u16 400, "MB session in"=w371) -> ("error out"=w363:errorcluster, "Coils"=w366:bool[], "MB session out"=w364:refnum<class "MB_Master.lvclass">)  [unwired: 5 in]
        n168 = case shown="无错误" w363 {
          tunnel: w366 -> [w395 _]
          frame No Error {
            n169 = global write "COD内部交互全局.vi" "温度"(w395) -> ()
            "温度" <- w395
          }
          frame Error {
          }
        }
        n170 = call <vilib>:"Read Coils.vi"("error in (no error)"=w363, "quantity"=u16 20, "starting address"=u16 500, "MB session in"=w364) -> ("error out"=w359:errorcluster, "Coils"=w358:bool[], "MB session out"=w362:refnum<class "MB_Master.lvclass">)  [unwired: 5 in]
        n171 = case shown="无错误" w359 {
          tunnel: w358 -> [w394 _]
          frame No Error {
            n172 = global write "COD内部交互全局.vi" "报警点位"(w394) -> ()
          }
          frame Error {
          }
        }
        n173 = Unbundle By Name(w359) -> ("status"=w343:bool)
        n174 = Not(x=w343) -> (.not. x?=w365:bool)
        "通讯状态" <- w365
        n175 = call <vilib>:"Boolean Crossing PtByPt.vi"("direction"=enum16{"either", "false-true", "true-false"}."either", "input"=w343) -> ("crossing"=w344:bool)  [unwired: 1 in]
        n176 = global write "COD内部交互全局.vi" "通讯状态"(w365) -> ()
        n177 = case shown="真" w344 {
          tunnel: w343 -> [_ w387]
          frame False {
          }
          frame True {
            n178 = case shown="真" w387 {
              tunnel: ["0" "999"] -> w386
              frame False {
              }
              frame True {
              }
            }
            n179 = Bundle By Name(cluster=T7 {"name"="", "CN"="", "FirmwareVersion"="", "code"=""} ("map in"), "name"="CODMn" ("componentParent"), "FirmwareVersion"="V1" ("ver"), "code"=w386) -> (w384:T7)
            n180 = call "告警接口-告警存储-交互.vi"("map in"=w384) -> ()  [unwired: 10 in, 1 out]
          }
        }
      }
      frame "CODMn读取写入DATABASE" {
        n181 = call <vilib>:"Read Holding Registers.vi"("error in (no error)"=w402, "quantity"=u16 10 ("number of holding registers"), "starting address"=u16 4101, "MB session in"=w405) -> ("error out"=w399:errorcluster, "Registers"=w400:u16[], "MB session out"=w401:refnum<class "MB_Master.lvclass">)  [unwired: 5 in]
        n182 = case shown="无错误" w399 {
          tunnel: w400 -> [w407 _]
          frame No Error {
            n183 = global write "COD内部交互全局.vi" "读取写入data"(TRUE ("读取参数显示")) -> ()
            n184 = global write "COD内部交互全局.vi" "数据存储"(w407) -> ()
            "数据存储" <- w407
          }
          frame Error {
          }
        }
      }
      frame "CODMn读取参数" {
        n185 = call <vilib>:"Read Holding Registers.vi"("error in (no error)"=w418, "quantity"=u16 65 ("number of holding registers"), "starting address"=u16 4272, "MB session in"=w419) -> ("error out"=w413:errorcluster, "Registers"=w415:u16[], "MB session out"=w414:refnum<class "MB_Master.lvclass">)  [unwired: 5 in]
        n186 = case shown="无错误" w413 {
          tunnel: w415 -> [w423 _]
          frame No Error {
            n187 = global write "COD内部交互全局.vi" "读取参数显示"(TRUE ("读取参数显示")) -> ()
            n188 = global write "COD内部交互全局.vi" "读取参数"(w423) -> ()
            "读取参数" <- w423
          }
          frame Error {
          }
        }
        n189 = call <vilib>:"Read Holding Registers.vi"("error in (no error)"=w413, "quantity"=u16 4, "starting address"=u16 5596, "MB session in"=w414) -> ("error out"=w409:errorcluster, "Registers"=w408:u16[], "MB session out"=w410:refnum<class "MB_Master.lvclass">)  [unwired: 5 in]
        n190 = case shown="无错误" w409 {
          tunnel: w408 -> [w421 _]
          frame No Error {
            n191 = global write "COD内部交互全局.vi" "读取浮台参数"(w421) -> ()
            n192 = global write "COD内部交互全局.vi" "读取浮台参数显示"(TRUE ("读取参数显示")) -> ()
          }
          frame Error {
          }
        }
      }
      frame "CODMn读取公式" {
        n193 = call <vilib>:"Read Holding Registers.vi"("error in (no error)"=w429, "quantity"=u16 94 ("number of holding registers"), "starting address"=u16 4616, "MB session in"=w430) -> ("error out"=w426:errorcluster, "Registers"=w428:u16[], "MB session out"=w427:refnum<class "MB_Master.lvclass">)  [unwired: 5 in]
        n194 = case shown="无错误" w426 {
          tunnel: w428 -> [w432 _]
          frame No Error {
            n195 = global write "COD内部交互全局.vi" "读取公式显示"(TRUE ("读取参数显示")) -> ()
            n196 = global write "COD内部交互全局.vi" "读取公式"(w432) -> ()
            "读取公式" <- w432
          }
          frame Error {
          }
        }
      }
      frame "CODMn序列号写入" {
        n197 = global read "COD内部交互全局.vi" "序列号:"() -> (w436:string)
        n198 = call "StringToHex.vi"("STRING"=w436) -> ("数组"=w435:u16[])  [unwired: 10 in]
        n199 = call <vilib>:"Write Multiple Registers.vi"("error in (no error)"=w437, "values"=w435, "starting address"=u16 4298, "MB session in"=w438) -> ("error out"=w433:errorcluster, "MB session out"=w434:refnum<class "MB_Master.lvclass">)  [unwired: 6 in]
      }
      frame "CODMn程序更新" {
        n200 = call <vilib>:"Write Multiple Registers.vi"("error in (no error)"=w442, "values"=u16[] [0], "starting address"=u16 4296, "MB session in"=w444) -> ("error out"=w440:errorcluster, "MB session out"=w441:refnum<class "MB_Master.lvclass">)  [unwired: 6 in]
      }
    }
  }
  n201 = Release Queue(queue=w4, error in (no error)=w3) -> ()  [unwired: 1 in, 3 out]
  n202 = Release Queue(queue=w9, error in (no error)=w8) -> ()  [unwired: 1 in, 3 out]
